vi "Get Specific Item Path.vi"(8 "error in (no error)":errorcluster, 9 "Item to find":string, 10 "Names":string[](array[string]), 11 "Decendant References":refnum<vi>[](array[refnum])) -> (0 "error out":errorcluster, 1 "Item Name":string, 2 "Item Path":path, 3 "Item Reference":refnum<vi>)   [LabVIEW 2015, in "Generic Module Library.lvlib"]
uses:
  Generic Module Library.lvlib
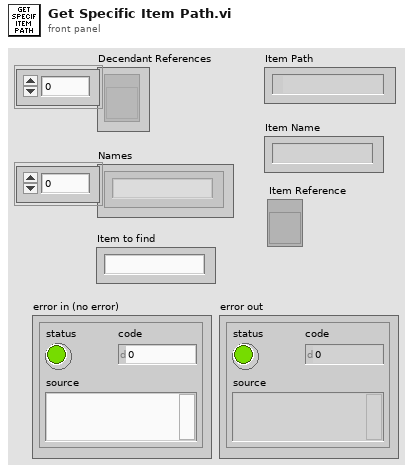
[diagram p1: front panel]
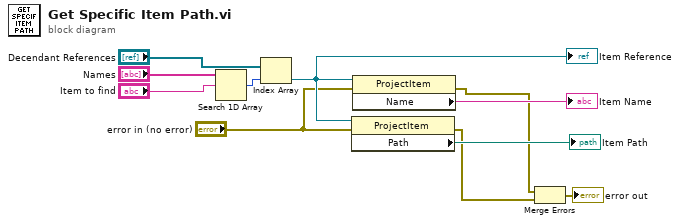
[diagram p0: block diagram]
diagram:
  n1 = Search 1D Array(1D array="Names", element="Item to find") -> (index of element=w7:i32)  [unwired: 1 in]
  n2 = Index Array(array="Decendant References", index=w7) -> (element=w10:refnum<vi>)
  "Item Reference" <- w10
  n3 = property class="ProjectItem"(reference=w10, error in="error in (no error)") -> (error out=w2:errorcluster, "Path"=→"Item Path":path)  [unwired: 1 out]
  n4 = property class="ProjectItem"(reference=w10, error in="error in (no error)") -> (error out=w3:errorcluster, "Name"=→"Item Name":string)  [unwired: 1 out]
  n5 = Merge Errors(w3, w2) -> (→"error out":errorcluster)
